vi "Destroy.vi"(0 "reference in":refnum<class "LightingSystem.lvclass">, 5 "Error In":errorcluster) -> (14 "reference out":refnum<class "LightingSystem.lvclass">, 19 "Error Out":errorcluster)   [LabVIEW 2024, in "LightingSystem.lvclass"]
uses:
  LightingSystem.lvclass/LightingSystem.ctl
  LightingSystem.lvclass
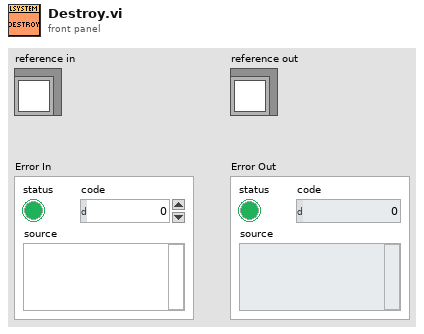
[diagram p1: front panel]
types:
  T1 = typedef "VI-TechBaseTemplate_Simple_6x8x6.lvclass/ObjectAttributes.ctl" = cluster{"Attribute1":dbl}
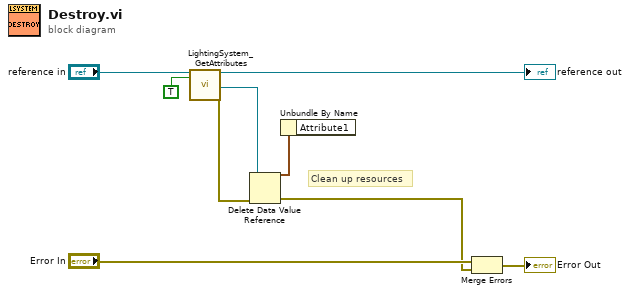
[diagram p0: block diagram]
diagram:
  # "Clean up resources"
  n1 = call "LightingSystem_GetAttributes.vi"("reference in"="reference in", "OnlyGetDvrReference(False)"=TRUE) -> ("reference out"=→"reference out":refnum<class "LightingSystem.lvclass">, "DataRef"=w5:refnum<data-value>, "Error Out"=w6:errorcluster)  [unwired: 14 in, 1 out]
  n2 = Delete Data Value Reference(data value reference=w5, error in=w6) -> (data value=w1:T1, error out=w3:errorcluster)
  n3 = Unbundle By Name(w1) -> ()  [unwired: 1 out]
  n4 = Merge Errors("Error In", w3) -> (→"Error Out":errorcluster)
